vi "main(Test DQMH modules).vi"() -> ()   [LabVIEW 2018, in "Application.lvlib"] (continued)
        n1221 = Build Array("Test DRV 31", "Test DRV 32", "Test DRV 33", "Test DRV 34", "Test DRV 35", "Test DRV 36", "MEAS.requestAC") -> (w2868:string[])
        n1222 = Reverse 1D Array(array=w2868) -> (reversed array=w2869:string[])
        n1223 = for {
          tunnel: w2869 -> [w2903] mode=indexing
          tunnel: [w2902] -> w2860 mode=indexing
          shift-right: [w2901] -> w2862
          shift-left: w2863 -> [w2904]
          tunnel: w2852 -> [w2900]
          n1224 = call "App enquece.vi"("Priority Enquece"=TRUE, "error in (no error)"=w2900, "command"=w2903, "queue in"=w2904) -> ("error out"=w2902:errorcluster, "Queue out"=w2901:refnum<queue>)  [unwired: 6 in]
        }
        n1225 = Initialize Array(TRUE, 6 ("dimension size")) -> (w2880:bool[])
        n1226 = Merge Errors(w2860) -> (w2859:errorcluster)
        n1227 = To Variant(anything=T5."mux10_1_channel6" ("mux10_1(x6)_encode")) -> (Variant=w2889:variant)
        n1228 = To Variant(anything=T6."demux1_10_channel6" ("demux1_10(x6)_encode")) -> (Variant=w2885:variant)
        n1229 = To Variant(anything=w2880) -> (Variant=w2879:variant)
        n1230 = Bundle By Name(cluster=w2877, "command"="MEAS.mux10-1", "command data"=w2889) -> (w2884:T11)
        n1231 = Bundle By Name(cluster=w2877, "command"="MEAS.demux1-10", "command data"=w2885) -> (w2883:T11)
        n1232 = Bundle By Name(cluster=w2877, "command"="MEAS.eMIC", "command data"=w2879) -> (w2878:T11)
        n1233 = Build Array(w2884, w2883, w2878) -> (w2858:T11[])
        n1234 = Reverse 1D Array(array=w2858) -> (reversed array=w2857:T11[])
        n1235 = for {
          tunnel: w2857 -> [w2915] mode=indexing
          tunnel: [w2912] -> w2870 mode=indexing
          tunnel: w2859 -> [w2911]
          tunnel: w2862 -> [w2916]
          n1236 = Unbundle By Name(w2915) -> ("command"=w2914:string, "command data"=w2913:variant)
          n1237 = call "App enquece.vi"("Priority Enquece"=TRUE, "error in (no error)"=w2911, "command data"=w2913, "command"=w2914, "queue in"=w2916) -> ("error out"=w2912:errorcluster)  [unwired: 5 in, 1 out]
        }
        n1238 = Merge Errors(w2873, w2870) -> (w2874:errorcluster)
      }
      frame "Test Channel 7" {
        w2947 = 7  # DUT channel (1-11)
        w2948 = T11 {"command"="", "command data"=variant} ("element")
        n1239 = disable-structure shown="LOGGING==TRUE" {
          disable-tunnel: w2942 -> [w2977 _]
          frame condition #0 (active) {
            n1240 = Empty String/Path?(string/path=w2977) -> (empty?=w2980:bool)
            n1241 = Select(t="Quece timeout", s=w2980, f=w2977) -> (s? t:f=w2976:string)
            n1242 = call "string log (SubVI).vi"("Enum"=enum16{"Init", "Log", "Read"}."Log", "state Name"=w2976) -> ()  [unwired: 8 in, 2 out]
          }
          frame condition #1 {
          }
        }
        n1243 = Build Array("Apps.UI Update", "MEAS.AllRelaysOFF2", "Apps.WaitForEvent") -> (w2926:string[])
        n1244 = for {
          tunnel: [w2967] -> w2933 mode=indexing
          shift-right: [w2968] -> w2934
          shift-left: w2929 -> [w2966]
          tunnel: w2926 -> [w2965] mode=indexing
          n1245 = call "App enquece.vi"("Priority Enquece"=TRUE, "command"=w2965, "queue in"=w2966) -> ("error out"=w2967:errorcluster, "Queue out"=w2968:refnum<queue>)  [unwired: 7 in]
        }
        n1246 = Merge Errors(w2933) -> (w2925:errorcluster)
        n1247 = Build Array("Test DRV 37", "Test DRV 38", "Test DRV 39", "Test DRV 40", "Test DRV 41", "Test DRV 42", "MEAS.requestAC") -> (w2939:string[])
        n1248 = Reverse 1D Array(array=w2939) -> (reversed array=w2940:string[])
        n1249 = for {
          tunnel: w2940 -> [w2974] mode=indexing
          tunnel: [w2973] -> w2932 mode=indexing
          shift-right: [w2972] -> w2924
          shift-left: w2934 -> [w2975]
          tunnel: w2925 -> [w2971]
          n1250 = call "App enquece.vi"("Priority Enquece"=TRUE, "error in (no error)"=w2971, "command"=w2974, "queue in"=w2975) -> ("error out"=w2973:errorcluster, "Queue out"=w2972:refnum<queue>)  [unwired: 6 in]
        }
        n1251 = Merge Errors(w2932) -> (w2931:errorcluster)
        n1252 = Initialize Array(TRUE, 6 ("dimension size")) -> (w2951:bool[])
        n1253 = To Variant(anything=w2951) -> (Variant=w2950:variant)
        n1254 = To Variant(anything=T5."mux10_1_channel7" ("mux10_1(x6)_encode")) -> (Variant=w2960:variant)
        n1255 = To Variant(anything=T6."demux1_10_channel7" ("demux1_10(x6)_encode")) -> (Variant=w2956:variant)
        n1256 = Bundle By Name(cluster=w2948, "command"="MEAS.mux10-1", "command data"=w2960) -> (w2955:T11)
        n1257 = Bundle By Name(cluster=w2948, "command"="MEAS.demux1-10", "command data"=w2956) -> (w2954:T11)
        n1258 = Bundle By Name(cluster=w2948, "command"="MEAS.eMIC", "command data"=w2950) -> (w2949:T11)
        n1259 = Build Array(w2955, w2954, w2949) -> (w2930:T11[])
        n1260 = Reverse 1D Array(array=w2930) -> (reversed array=w2923:T11[])
        n1261 = for {
          tunnel: w2923 -> [w2987] mode=indexing
          tunnel: [w2984] -> w2941 mode=indexing
          tunnel: w2931 -> [w2983]
          tunnel: w2924 -> [w2981]
          n1262 = Unbundle By Name(w2987) -> ("command"=w2986:string, "command data"=w2985:variant)
          n1263 = call "App enquece.vi"("Priority Enquece"=TRUE, "error in (no error)"=w2983, "command data"=w2985, "command"=w2986, "queue in"=w2981) -> ("error out"=w2984:errorcluster)  [unwired: 5 in, 1 out]
        }
        n1264 = Merge Errors(w2944, w2941) -> (w2945:errorcluster)
      }
      frame "Test Channel 8" {
        w3018 = 8  # DUT channel (1-11)
        w3019 = T11 {"command"="", "command data"=variant} ("element")
        n1265 = disable-structure shown="LOGGING==TRUE" {
          disable-tunnel: w3013 -> [w3048 _]
          frame condition #0 (active) {
            n1266 = Empty String/Path?(string/path=w3048) -> (empty?=w3051:bool)
            n1267 = Select(t="Quece timeout", s=w3051, f=w3048) -> (s? t:f=w3047:string)
            n1268 = call "string log (SubVI).vi"("Enum"=enum16{"Init", "Log", "Read"}."Log", "state Name"=w3047) -> ()  [unwired: 8 in, 2 out]
          }
          frame condition #1 {
          }
        }
        n1269 = Build Array("Apps.UI Update", "MEAS.AllRelaysOFF2", "Apps.WaitForEvent") -> (w2997:string[])
        n1270 = for {
          tunnel: [w3038] -> w3005 mode=indexing
          shift-right: [w3039] -> w3007
          shift-left: w3000 -> [w3037]
          tunnel: w2997 -> [w3036] mode=indexing
          n1271 = call "App enquece.vi"("Priority Enquece"=TRUE, "command"=w3036, "queue in"=w3037) -> ("error out"=w3038:errorcluster, "Queue out"=w3039:refnum<queue>)  [unwired: 7 in]
        }
        n1272 = Merge Errors(w3005) -> (w2996:errorcluster)
        n1273 = Build Array("Test DRV 43", "Test DRV 44", "Test DRV 45", "Test DRV 46", "Test DRV 47", "Test DRV 48", "MEAS.requestAC") -> (w3010:string[])
        n1274 = Reverse 1D Array(array=w3010) -> (reversed array=w3011:string[])
        n1275 = for {
          tunnel: w3011 -> [w3045] mode=indexing
          tunnel: [w3044] -> w3004 mode=indexing
          shift-right: [w3043] -> w3006
          shift-left: w3007 -> [w3046]
          tunnel: w2996 -> [w3042]
          n1276 = call "App enquece.vi"("Priority Enquece"=TRUE, "error in (no error)"=w3042, "command"=w3045, "queue in"=w3046) -> ("error out"=w3044:errorcluster, "Queue out"=w3043:refnum<queue>)  [unwired: 6 in]
        }
        n1277 = Initialize Array(TRUE, 6 ("dimension size")) -> (w3022:bool[])
        n1278 = Merge Errors(w3004) -> (w3003:errorcluster)
        n1279 = To Variant(anything=T5."mux10_1_channel8" ("mux10_1(x6)_encode")) -> (Variant=w3031:variant)
        n1280 = To Variant(anything=T6."demux1_10_channel8" ("demux1_10(x6)_encode")) -> (Variant=w3027:variant)
        n1281 = To Variant(anything=w3022) -> (Variant=w3021:variant)
        n1282 = Bundle By Name(cluster=w3019, "command"="MEAS.mux10-1", "command data"=w3031) -> (w3026:T11)
        n1283 = Bundle By Name(cluster=w3019, "command"="MEAS.demux1-10", "command data"=w3027) -> (w3025:T11)
        n1284 = Bundle By Name(cluster=w3019, "command"="MEAS.eMIC", "command data"=w3021) -> (w3020:T11)
        n1285 = Build Array(w3026, w3025, w3020) -> (w3002:T11[])
        n1286 = Reverse 1D Array(array=w3002) -> (reversed array=w3001:T11[])
        n1287 = for {
          tunnel: w3001 -> [w3057] mode=indexing
          tunnel: [w3054] -> w3012 mode=indexing
          tunnel: w3003 -> [w3053]
          tunnel: w3006 -> [w3058]
          n1288 = Unbundle By Name(w3057) -> ("command"=w3056:string, "command data"=w3055:variant)
          n1289 = call "App enquece.vi"("Priority Enquece"=TRUE, "error in (no error)"=w3053, "command data"=w3055, "command"=w3056, "queue in"=w3058) -> ("error out"=w3054:errorcluster)  [unwired: 5 in, 1 out]
        }
        n1290 = Merge Errors(w3015, w3012) -> (w3016:errorcluster)
      }
      frame "Test Channel 9" {
        w3090 = 9  # DUT channel (1-10)
        w3091 = T11 {"command"="", "command data"=variant} ("element")
        n1291 = disable-structure shown="LOGGING==TRUE" {
          disable-tunnel: w3085 -> [w3119 _]
          frame condition #0 (active) {
            n1292 = Empty String/Path?(string/path=w3119) -> (empty?=w3122:bool)
            n1293 = Select(t="Quece timeout", s=w3122, f=w3119) -> (s? t:f=w3118:string)
            n1294 = call "string log (SubVI).vi"("Enum"=enum16{"Init", "Log", "Read"}."Log", "state Name"=w3118) -> ()  [unwired: 8 in, 2 out]
          }
          frame condition #1 {
          }
        }
        n1295 = Build Array("Apps.UI Update", "MEAS.AllRelaysOFF2", "Apps.WaitForEvent") -> (w3067:string[])
        n1296 = for {
          tunnel: [w3109] -> w3076 mode=indexing
          shift-right: [w3110] -> w3078
          shift-left: w3071 -> [w3108]
          tunnel: w3067 -> [w3107] mode=indexing
          n1297 = call "App enquece.vi"("Priority Enquece"=TRUE, "command"=w3107, "queue in"=w3108) -> ("error out"=w3109:errorcluster, "Queue out"=w3110:refnum<queue>)  [unwired: 7 in]
        }
        n1298 = Merge Errors(w3076) -> (w3066:errorcluster)
        n1299 = Build Array("Test DRV 49", "Test DRV 50", "Test DRV 51", "Test DRV 52", "Test DRV 53", "Test DRV 54", "MEAS.requestAC") -> (w3082:string[])
        n1300 = Reverse 1D Array(array=w3082) -> (reversed array=w3083:string[])
        n1301 = for {
          tunnel: w3083 -> [w3116] mode=indexing
          tunnel: [w3115] -> w3075 mode=indexing
          shift-right: [w3114] -> w3077
          shift-left: w3078 -> [w3117]
          tunnel: w3066 -> [w3113]
          n1302 = call "App enquece.vi"("Priority Enquece"=TRUE, "error in (no error)"=w3113, "command"=w3116, "queue in"=w3117) -> ("error out"=w3115:errorcluster, "Queue out"=w3114:refnum<queue>)  [unwired: 6 in]
        }
        n1303 = Merge Errors(w3075) -> (w3074:errorcluster)
        n1304 = Initialize Array(TRUE, 6 ("dimension size")) -> (w3094:bool[])
        n1305 = To Variant(anything=T5."mux10_1_channel9" ("mux10_1(x6)_encode")) -> (Variant=w3103:variant)
        n1306 = To Variant(anything=T6."demux1_10_channel9" ("demux1_10(x6)_encode")) -> (Variant=w3099:variant)
        n1307 = To Variant(anything=w3094) -> (Variant=w3093:variant)
        n1308 = Bundle By Name(cluster=w3091, "command"="MEAS.mux10-1", "command data"=w3103) -> (w3098:T11)
        n1309 = Bundle By Name(cluster=w3091, "command"="MEAS.demux1-10", "command data"=w3099) -> (w3097:T11)
        n1310 = Bundle By Name(cluster=w3091, "command"="MEAS.eMIC", "command data"=w3093) -> (w3092:T11)
        n1311 = Build Array(w3098, w3097, w3092) -> (w3073:T11[])
        n1312 = Reverse 1D Array(array=w3073) -> (reversed array=w3072:T11[])
        n1313 = for {
          tunnel: w3072 -> [w3128] mode=indexing
          tunnel: [w3125] -> w3084 mode=indexing
          tunnel: w3074 -> [w3124]
          tunnel: w3077 -> [w3129]
          n1314 = Unbundle By Name(w3128) -> ("command"=w3127:string, "command data"=w3126:variant)
          n1315 = call "App enquece.vi"("Priority Enquece"=TRUE, "error in (no error)"=w3124, "command data"=w3126, "command"=w3127, "queue in"=w3129) -> ("error out"=w3125:errorcluster)  [unwired: 5 in, 1 out]
        }
        n1316 = Merge Errors(w3087, w3084) -> (w3088:errorcluster)
      }
      frame "Test Channel 10" {
        w3163 = 10  # DUT channel (1-10)
        w3139 = T11 {"command"="", "command data"=variant} ("element")
        n1317 = disable-structure shown="LOGGING==TRUE" {
          disable-tunnel: w3158 -> [w3190 _]
          frame condition #0 (active) {
            n1318 = Empty String/Path?(string/path=w3190) -> (empty?=w3193:bool)
            n1319 = Select(t="Quece timeout", s=w3193, f=w3190) -> (s? t:f=w3189:string)
            n1320 = call "string log (SubVI).vi"("Enum"=enum16{"Init", "Log", "Read"}."Log", "state Name"=w3189) -> ()  [unwired: 8 in, 2 out]
          }
          frame condition #1 {
          }
        }
        n1321 = Build Array("Apps.UI Update", "MEAS.AllRelaysOFF2", "Apps.WaitForEvent") -> (w3141:string[])
        n1322 = for {
          tunnel: [w3180] -> w3149 mode=indexing
          shift-right: [w3181] -> w3151
          shift-left: w3144 -> [w3179]
          tunnel: w3141 -> [w3178] mode=indexing
          n1323 = call "App enquece.vi"("Priority Enquece"=TRUE, "command"=w3178, "queue in"=w3179) -> ("error out"=w3180:errorcluster, "Queue out"=w3181:refnum<queue>)  [unwired: 7 in]
        }
        n1324 = Merge Errors(w3149) -> (w3140:errorcluster)
        n1325 = Build Array("Test DRV 55", "Test DRV 56", "Test DRV 57", "Test DRV 58", "Test DRV 59", "Test DRV 60", "MEAS.requestAC") -> (w3155:string[])
        n1326 = Reverse 1D Array(array=w3155) -> (reversed array=w3156:string[])
        n1327 = for {
          tunnel: w3156 -> [w3187] mode=indexing
          tunnel: [w3186] -> w3148 mode=indexing
          shift-right: [w3185] -> w3150
          shift-left: w3151 -> [w3188]
          tunnel: w3140 -> [w3184]
          n1328 = call "App enquece.vi"("Priority Enquece"=TRUE, "error in (no error)"=w3184, "command"=w3187, "queue in"=w3188) -> ("error out"=w3186:errorcluster, "Queue out"=w3185:refnum<queue>)  [unwired: 6 in]
        }
        n1329 = Initialize Array(TRUE, 6 ("dimension size")) -> (w3133:bool[])
        n1330 = To Variant(anything=w3133) -> (Variant=w3165:variant)
        n1331 = To Variant(anything=T5."mux10_1_channel10" ("mux10_1(x6)_encode")) -> (Variant=w3173:variant)
        n1332 = To Variant(anything=T6."demux1_10_channel10" ("demux1_10(x6)_encode")) -> (Variant=w3169:variant)
        n1333 = Bundle By Name(cluster=w3139, "command"="MEAS.mux10-1", "command data"=w3173) -> (w3168:T11)
        n1334 = Bundle By Name(cluster=w3139, "command"="MEAS.demux1-10", "command data"=w3169) -> (w3167:T11)
        n1335 = Bundle By Name(cluster=w3139, "command"="MEAS.eMIC", "command data"=w3165) -> (w3164:T11)
        n1336 = Merge Errors(w3148) -> (w3147:errorcluster)
        n1337 = Build Array(w3168, w3167, w3164) -> (w3146:T11[])
        n1338 = Reverse 1D Array(array=w3146) -> (reversed array=w3145:T11[])
        n1339 = for {
          tunnel: w3145 -> [w3199] mode=indexing
          tunnel: [w3196] -> w3157 mode=indexing
          tunnel: w3147 -> [w3195]
          tunnel: w3150 -> [w3200]
          n1340 = Unbundle By Name(w3199) -> ("command"=w3198:string, "command data"=w3197:variant)
          n1341 = call "App enquece.vi"("Priority Enquece"=TRUE, "error in (no error)"=w3195, "command data"=w3197, "command"=w3198, "queue in"=w3200) -> ("error out"=w3196:errorcluster)  [unwired: 5 in, 1 out]
        }
        n1342 = Merge Errors(w3160, w3157) -> (w3161:errorcluster)
      }
      frame "Test Channel 10A" {
        w3211 = T11 {"command"="", "command data"=variant} ("element")
        w3239 = 10  # DUT channel (1-10)
        w3219 = T11 {"command"="", "command data"=variant} ("element")
        n1343 = disable-structure shown="LOGGING==TRUE" {
          disable-tunnel: w3234 -> [w3268 _]
          frame condition #0 (active) {
            n1344 = Empty String/Path?(string/path=w3268) -> (empty?=w3271:bool)
            n1345 = Select(t="Quece timeout", s=w3271, f=w3268) -> (s? t:f=w3267:string)
            n1346 = call "string log (SubVI).vi"("Enum"=enum16{"Init", "Log", "Read"}."Log", "state Name"=w3267) -> ()  [unwired: 8 in, 2 out]
          }
          frame condition #1 {
          }
        }
        n1347 = Bundle By Name(cluster=w3211, "command"="Apps.UI Update", "command data"="A") -> (w3210:T11)
        n1348 = Bundle By Name(cluster=w3211, "command"="MEAS.AllRelaysOFF2") -> (w3209:T11)
        n1349 = Bundle By Name(cluster=w3211, "command"="Apps.WaitForEvent") -> (w3208:T11)
        n1350 = Build Array(w3210, w3209, w3208) -> (w3221:T11[])
        n1351 = for {
          tunnel: [w3258] -> w3228 mode=indexing
          shift-right: [w3259] -> w3230
          shift-left: w3223 -> [w3257]
          tunnel: w3221 -> [w3256] mode=indexing
          n1352 = Unbundle By Name(w3256) -> ("command"=w3255:string, "command data"=w3254:variant)
          n1353 = call "App enquece.vi"("Priority Enquece"=TRUE, "command data"=w3254, "command"=w3255, "queue in"=w3257) -> ("error out"=w3258:errorcluster, "Queue out"=w3259:refnum<queue>)  [unwired: 6 in]
        }
        n1354 = Merge Errors(w3228) -> (w3220:errorcluster)
        n1355 = Build Array("Test DRV 55", "WaitFor", "MEAS.requestAC") -> (w3231:string[])
        n1356 = Reverse 1D Array(array=w3231) -> (reversed array=w3232:string[])
        n1357 = for {
          tunnel: w3232 -> [w3265] mode=indexing
          tunnel: [w3264] -> w3227 mode=indexing
          shift-right: [w3263] -> w3229
          shift-left: w3230 -> [w3266]
          tunnel: w3220 -> [w3262]
          n1358 = call "App enquece.vi"("Priority Enquece"=TRUE, "error in (no error)"=w3262, "command"=w3265, "queue in"=w3266) -> ("error out"=w3264:errorcluster, "Queue out"=w3263:refnum<queue>)  [unwired: 6 in]
        }
        n1359 = Initialize Array(FALSE ("element"), 6 ("dimension size")) -> (w3205:bool[])
        n1360 = Initialize Array(TRUE, 1 ("dimension size")) -> (w3204:bool[])
        n1361 = Replace Array Subset(array=w3205, new element=w3204) -> (w3203:bool[])  [unwired: 1 in]
        n1362 = To Variant(anything=T5."mux10_1_channel10" ("mux10_1(x6)_encode")) -> (Variant=w3249:variant)
        n1363 = To Variant(anything=T6."demux1_10_channel10" ("demux1_10(x6)_encode")) -> (Variant=w3245:variant)
        n1364 = To Variant(anything=w3203) -> (Variant=w3241:variant)
        n1365 = Merge Errors(w3227) -> (w3226:errorcluster)
        n1366 = Bundle By Name(cluster=w3219, "command"="MEAS.mux10-1", "command data"=w3249) -> (w3244:T11)
        n1367 = Bundle By Name(cluster=w3219, "command"="MEAS.demux1-10", "command data"=w3245) -> (w3243:T11)
        n1368 = Bundle By Name(cluster=w3219, "command"="MEAS.eMIC", "command data"=w3241) -> (w3240:T11)
        n1369 = Build Array(w3244, w3243, w3240) -> (w3225:T11[])
        n1370 = Reverse 1D Array(array=w3225) -> (reversed array=w3224:T11[])
        n1371 = for {
          tunnel: w3224 -> [w3277] mode=indexing
          tunnel: [w3274] -> w3233 mode=indexing
          tunnel: w3226 -> [w3273]
          tunnel: w3229 -> [w3278]
          n1372 = Unbundle By Name(w3277) -> ("command"=w3276:string, "command data"=w3275:variant)
          n1373 = call "App enquece.vi"("Priority Enquece"=TRUE, "error in (no error)"=w3273, "command data"=w3275, "command"=w3276, "queue in"=w3278) -> ("error out"=w3274:errorcluster)  [unwired: 5 in, 1 out]
        }
        n1374 = Merge Errors(w3236, w3233) -> (w3237:errorcluster)
      }
      frame "Test Channel 10B" {
        w3289 = T11 {"command"="", "command data"=variant} ("element")
        w3318 = 10  # DUT channel (1-10)
        w3297 = T11 {"command"="", "command data"=variant} ("element")
        n1375 = disable-structure shown="LOGGING==TRUE" {
          disable-tunnel: w3313 -> [w3347 _]
          frame condition #0 (active) {
            n1376 = Empty String/Path?(string/path=w3347) -> (empty?=w3350:bool)
            n1377 = Select(t="Quece timeout", s=w3350, f=w3347) -> (s? t:f=w3346:string)
            n1378 = call "string log (SubVI).vi"("Enum"=enum16{"Init", "Log", "Read"}."Log", "state Name"=w3346) -> ()  [unwired: 8 in, 2 out]
          }
          frame condition #1 {
          }
        }
        n1379 = Bundle By Name(cluster=w3289, "command"="Apps.UI Update", "command data"="B") -> (w3288:T11)
        n1380 = Bundle By Name(cluster=w3289, "command"="MEAS.AllRelaysOFF2") -> (w3287:T11)
        n1381 = Bundle By Name(cluster=w3289, "command"="Apps.WaitForEvent") -> (w3286:T11)
        n1382 = Build Array(w3288, w3287, w3286) -> (w3299:T11[])
        n1383 = for {
          tunnel: [w3337] -> w3306 mode=indexing
          shift-right: [w3338] -> w3308
          shift-left: w3301 -> [w3336]
          tunnel: w3299 -> [w3335] mode=indexing
          n1384 = Unbundle By Name(w3335) -> ("command"=w3334:string, "command data"=w3333:variant)
          n1385 = call "App enquece.vi"("Priority Enquece"=TRUE, "command data"=w3333, "command"=w3334, "queue in"=w3336) -> ("error out"=w3337:errorcluster, "Queue out"=w3338:refnum<queue>)  [unwired: 6 in]
        }
        n1386 = Merge Errors(w3306) -> (w3298:errorcluster)
        n1387 = Build Array("Test DRV 55", "Test DRV 56", "WaitFor", "MEAS.requestAC") -> (w3310:string[])
        n1388 = Reverse 1D Array(array=w3310) -> (reversed array=w3311:string[])
        n1389 = for {
          tunnel: w3311 -> [w3344] mode=indexing
          tunnel: [w3343] -> w3305 mode=indexing
          shift-right: [w3342] -> w3307
          shift-left: w3308 -> [w3345]
          tunnel: w3298 -> [w3341]
          n1390 = call "App enquece.vi"("Priority Enquece"=TRUE, "error in (no error)"=w3341, "command"=w3344, "queue in"=w3345) -> ("error out"=w3343:errorcluster, "Queue out"=w3342:refnum<queue>)  [unwired: 6 in]
        }
        n1391 = Initialize Array(FALSE ("element"), 6 ("dimension size")) -> (w3281:bool[])
        n1392 = Initialize Array(TRUE, 2 ("dimension size")) -> (w3280:bool[])
        n1393 = Replace Array Subset(array=w3281, new element=w3280) -> (w3279:bool[])  [unwired: 1 in]
        n1394 = To Variant(anything=T5."mux10_1_channel10" ("mux10_1(x6)_encode")) -> (Variant=w3328:variant)
        n1395 = To Variant(anything=T6."demux1_10_channel10" ("demux1_10(x6)_encode")) -> (Variant=w3324:variant)
        n1396 = To Variant(anything=w3279) -> (Variant=w3320:variant)
        n1397 = Merge Errors(w3305) -> (w3304:errorcluster)
        n1398 = Bundle By Name(cluster=w3297, "command"="MEAS.mux10-1", "command data"=w3328) -> (w3323:T11)
        n1399 = Bundle By Name(cluster=w3297, "command"="MEAS.demux1-10", "command data"=w3324) -> (w3322:T11)
        n1400 = Bundle By Name(cluster=w3297, "command"="MEAS.eMIC", "command data"=w3320) -> (w3319:T11)
        n1401 = Build Array(w3323, w3322, w3319) -> (w3303:T11[])
        n1402 = Reverse 1D Array(array=w3303) -> (reversed array=w3302:T11[])
        n1403 = for {
          tunnel: w3302 -> [w3356] mode=indexing
          tunnel: [w3353] -> w3312 mode=indexing
          tunnel: w3304 -> [w3352]
          tunnel: w3307 -> [w3357]
          n1404 = Unbundle By Name(w3356) -> ("command"=w3355:string, "command data"=w3354:variant)
          n1405 = call "App enquece.vi"("Priority Enquece"=TRUE, "error in (no error)"=w3352, "command data"=w3354, "command"=w3355, "queue in"=w3357) -> ("error out"=w3353:errorcluster)  [unwired: 5 in, 1 out]
        }
        n1406 = Merge Errors(w3315, w3312) -> (w3316:errorcluster)
      }
      frame "Test Channel 10C" {
        w3371 = T11 {"command"="", "command data"=variant} ("element")
        w3398 = 10  # DUT channel (1-10)
        w3378 = T11 {"command"="", "command data"=variant} ("element")
        n1407 = disable-structure shown="LOGGING==TRUE" {
          disable-tunnel: w3393 -> [w3427 _]
          frame condition #0 (active) {
            n1408 = Empty String/Path?(string/path=w3427) -> (empty?=w3430:bool)
            n1409 = Select(t="Quece timeout", s=w3430, f=w3427) -> (s? t:f=w3426:string)
            n1410 = call "string log (SubVI).vi"("Enum"=enum16{"Init", "Log", "Read"}."Log", "state Name"=w3426) -> ()  [unwired: 8 in, 2 out]
          }
          frame condition #1 {
          }
        }
        n1411 = Bundle By Name(cluster=w3371, "command"="Apps.UI Update", "command data"="C") -> (w3370:T11)
        n1412 = Bundle By Name(cluster=w3371, "command"="MEAS.AllRelaysOFF2") -> (w3369:T11)
        n1413 = Bundle By Name(cluster=w3371, "command"="Apps.WaitForEvent") -> (w3368:T11)
        n1414 = Build Array(w3370, w3369, w3368) -> (w3380:T11[])
        n1415 = for {
          tunnel: [w3417] -> w3387 mode=indexing
          shift-right: [w3418] -> w3389
          shift-left: w3382 -> [w3416]
          tunnel: w3380 -> [w3415] mode=indexing
          n1416 = Unbundle By Name(w3415) -> ("command"=w3414:string, "command data"=w3413:variant)
          n1417 = call "App enquece.vi"("Priority Enquece"=TRUE, "command data"=w3413, "command"=w3414, "queue in"=w3416) -> ("error out"=w3417:errorcluster, "Queue out"=w3418:refnum<queue>)  [unwired: 6 in]
        }
        n1418 = Merge Errors(w3387) -> (w3379:errorcluster)
        n1419 = Build Array("Test DRV 55", "Test DRV 56", "Test DRV 57", "WaitFor", "MEAS.requestAC") -> (w3390:string[])
        n1420 = Reverse 1D Array(array=w3390) -> (reversed array=w3391:string[])
        n1421 = for {
          tunnel: w3391 -> [w3424] mode=indexing
          tunnel: [w3423] -> w3386 mode=indexing
          shift-right: [w3422] -> w3388
          shift-left: w3389 -> [w3425]
          tunnel: w3379 -> [w3421]
          n1422 = call "App enquece.vi"("Priority Enquece"=TRUE, "error in (no error)"=w3421, "command"=w3424, "queue in"=w3425) -> ("error out"=w3423:errorcluster, "Queue out"=w3422:refnum<queue>)  [unwired: 6 in]
        }
        n1423 = Initialize Array(FALSE ("element"), 6 ("dimension size")) -> (w3363:bool[])
        n1424 = Initialize Array(TRUE, 3 ("dimension size")) -> (w3362:bool[])
        n1425 = Replace Array Subset(array=w3363, new element=w3362) -> (w3361:bool[])  [unwired: 1 in]
        n1426 = To Variant(anything=T5."mux10_1_channel10" ("mux10_1(x6)_encode")) -> (Variant=w3408:variant)
        n1427 = To Variant(anything=T6."demux1_10_channel10" ("demux1_10(x6)_encode")) -> (Variant=w3404:variant)
        n1428 = To Variant(anything=w3361) -> (Variant=w3400:variant)
        n1429 = Merge Errors(w3386) -> (w3385:errorcluster)
        n1430 = Bundle By Name(cluster=w3378, "command"="MEAS.mux10-1", "command data"=w3408) -> (w3403:T11)
        n1431 = Bundle By Name(cluster=w3378, "command"="MEAS.demux1-10", "command data"=w3404) -> (w3402:T11)
        n1432 = Bundle By Name(cluster=w3378, "command"="MEAS.eMIC", "command data"=w3400) -> (w3399:T11)
        n1433 = Build Array(w3403, w3402, w3399) -> (w3384:T11[])
        n1434 = Reverse 1D Array(array=w3384) -> (reversed array=w3383:T11[])
        n1435 = for {
          tunnel: w3383 -> [w3436] mode=indexing
          tunnel: [w3433] -> w3392 mode=indexing
          tunnel: w3385 -> [w3432]
          tunnel: w3388 -> [w3437]
          n1436 = Unbundle By Name(w3436) -> ("command"=w3435:string, "command data"=w3434:variant)
          n1437 = call "App enquece.vi"("Priority Enquece"=TRUE, "error in (no error)"=w3432, "command data"=w3434, "command"=w3435, "queue in"=w3437) -> ("error out"=w3433:errorcluster)  [unwired: 5 in, 1 out]
        }
        n1438 = Merge Errors(w3395, w3392) -> (w3396:errorcluster)
      }
      frame "Test Channel 10D" {
        w3452 = T11 {"command"="", "command data"=variant} ("element")
        w3479 = 10  # DUT channel (1-10)
        w3459 = T11 {"command"="", "command data"=variant} ("element")
        n1439 = disable-structure shown="LOGGING==TRUE" {
          disable-tunnel: w3474 -> [w3508 _]
          frame condition #0 (active) {
            n1440 = Empty String/Path?(string/path=w3508) -> (empty?=w3511:bool)
            n1441 = Select(t="Quece timeout", s=w3511, f=w3508) -> (s? t:f=w3507:string)
            n1442 = call "string log (SubVI).vi"("Enum"=enum16{"Init", "Log", "Read"}."Log", "state Name"=w3507) -> ()  [unwired: 8 in, 2 out]
          }
          frame condition #1 {
          }
        }
        n1443 = Bundle By Name(cluster=w3452, "command"="Apps.UI Update", "command data"="D") -> (w3451:T11)
        n1444 = Bundle By Name(cluster=w3452, "command"="MEAS.AllRelaysOFF2") -> (w3450:T11)
        n1445 = Bundle By Name(cluster=w3452, "command"="Apps.WaitForEvent") -> (w3449:T11)
        n1446 = Build Array(w3451, w3450, w3449) -> (w3461:T11[])
        n1447 = for {
          tunnel: [w3498] -> w3468 mode=indexing
          shift-right: [w3499] -> w3470
          shift-left: w3463 -> [w3497]
          tunnel: w3461 -> [w3496] mode=indexing
          n1448 = Unbundle By Name(w3496) -> ("command"=w3495:string, "command data"=w3494:variant)
          n1449 = call "App enquece.vi"("Priority Enquece"=TRUE, "command data"=w3494, "command"=w3495, "queue in"=w3497) -> ("error out"=w3498:errorcluster, "Queue out"=w3499:refnum<queue>)  [unwired: 6 in]
        }
        n1450 = Merge Errors(w3468) -> (w3460:errorcluster)
        n1451 = Build Array("Test DRV 55", "Test DRV 56", "Test DRV 57", "Test DRV 58", "WaitFor", "MEAS.requestAC") -> (w3471:string[])
        n1452 = Reverse 1D Array(array=w3471) -> (reversed array=w3472:string[])
        n1453 = for {
          tunnel: w3472 -> [w3505] mode=indexing
          tunnel: [w3504] -> w3467 mode=indexing
          shift-right: [w3503] -> w3469
          shift-left: w3470 -> [w3506]
          tunnel: w3460 -> [w3502]
          n1454 = call "App enquece.vi"("Priority Enquece"=TRUE, "error in (no error)"=w3502, "command"=w3505, "queue in"=w3506) -> ("error out"=w3504:errorcluster, "Queue out"=w3503:refnum<queue>)  [unwired: 6 in]
        }
        n1455 = Initialize Array(FALSE ("element"), 6 ("dimension size")) -> (w3444:bool[])
        n1456 = Initialize Array(TRUE, 4 ("dimension size")) -> (w3443:bool[])
        n1457 = Replace Array Subset(array=w3444, new element=w3443) -> (w3442:bool[])  [unwired: 1 in]
        n1458 = To Variant(anything=T5."mux10_1_channel10" ("mux10_1(x6)_encode")) -> (Variant=w3489:variant)
        n1459 = To Variant(anything=T6."demux1_10_channel10" ("demux1_10(x6)_encode")) -> (Variant=w3485:variant)
        n1460 = To Variant(anything=w3442) -> (Variant=w3481:variant)
        n1461 = Merge Errors(w3467) -> (w3466:errorcluster)
        n1462 = Bundle By Name(cluster=w3459, "command"="MEAS.mux10-1", "command data"=w3489) -> (w3484:T11)
        n1463 = Bundle By Name(cluster=w3459, "command"="MEAS.demux1-10", "command data"=w3485) -> (w3483:T11)
        n1464 = Bundle By Name(cluster=w3459, "command"="MEAS.eMIC", "command data"=w3481) -> (w3480:T11)
        n1465 = Build Array(w3484, w3483, w3480) -> (w3465:T11[])
        n1466 = Reverse 1D Array(array=w3465) -> (reversed array=w3464:T11[])
        n1467 = for {
          tunnel: w3464 -> [w3517] mode=indexing
          tunnel: [w3514] -> w3473 mode=indexing
          tunnel: w3466 -> [w3513]
          tunnel: w3469 -> [w3518]
          n1468 = Unbundle By Name(w3517) -> ("command"=w3516:string, "command data"=w3515:variant)
          n1469 = call "App enquece.vi"("Priority Enquece"=TRUE, "error in (no error)"=w3513, "command data"=w3515, "command"=w3516, "queue in"=w3518) -> ("error out"=w3514:errorcluster)  [unwired: 5 in, 1 out]
        }
        n1470 = Merge Errors(w3476, w3473) -> (w3477:errorcluster)
      }
      frame "Test Channel 10E" {
        w3535 = T11 {"command"="", "command data"=variant} ("element")
        w3561 = 10  # DUT channel (1-10)
        w3542 = T11 {"command"="", "command data"=variant} ("element")
        n1471 = disable-structure shown="LOGGING==TRUE" {
          disable-tunnel: w3556 -> [w3590 _]
          frame condition #0 (active) {
            n1472 = Empty String/Path?(string/path=w3590) -> (empty?=w3593:bool)
            n1473 = Select(t="Quece timeout", s=w3593, f=w3590) -> (s? t:f=w3589:string)
            n1474 = call "string log (SubVI).vi"("Enum"=enum16{"Init", "Log", "Read"}."Log", "state Name"=w3589) -> ()  [unwired: 8 in, 2 out]
          }
          frame condition #1 {
          }
        }
        n1475 = Bundle By Name(cluster=w3535, "command"="Apps.UI Update", "command data"="E") -> (w3534:T11)
        n1476 = Bundle By Name(cluster=w3535, "command"="MEAS.AllRelaysOFF2") -> (w3533:T11)
        n1477 = Bundle By Name(cluster=w3535, "command"="Apps.WaitForEvent") -> (w3532:T11)
        n1478 = Build Array(w3534, w3533, w3532) -> (w3544:T11[])
        n1479 = for {
          tunnel: [w3580] -> w3551 mode=indexing
          shift-right: [w3581] -> w3553
          shift-left: w3546 -> [w3579]
          tunnel: w3544 -> [w3578] mode=indexing
          n1480 = Unbundle By Name(w3578) -> ("command"=w3577:string, "command data"=w3576:variant)
          n1481 = call "App enquece.vi"("Priority Enquece"=TRUE, "command data"=w3576, "command"=w3577, "queue in"=w3579) -> ("error out"=w3580:errorcluster, "Queue out"=w3581:refnum<queue>)  [unwired: 6 in]
        }
        n1482 = Merge Errors(w3551) -> (w3543:errorcluster)
        n1483 = Build Array("Test DRV 55", "Test DRV 56", "Test DRV 57", "Test DRV 58", "Test DRV 59", "WaitFor", "MEAS.requestAC") -> (w3519:string[])
        n1484 = Reverse 1D Array(array=w3519) -> (reversed array=w3554:string[])
        n1485 = for {
          tunnel: w3554 -> [w3587] mode=indexing
          tunnel: [w3586] -> w3550 mode=indexing
          shift-right: [w3585] -> w3552
          shift-left: w3553 -> [w3588]
          tunnel: w3543 -> [w3584]
          n1486 = call "App enquece.vi"("Priority Enquece"=TRUE, "error in (no error)"=w3584, "command"=w3587, "queue in"=w3588) -> ("error out"=w3586:errorcluster, "Queue out"=w3585:refnum<queue>)  [unwired: 6 in]
        }
        n1487 = Initialize Array(FALSE ("element"), 6 ("dimension size")) -> (w3529:bool[])
        n1488 = Initialize Array(TRUE, 5 ("dimension size")) -> (w3528:bool[])
        n1489 = Replace Array Subset(array=w3529, new element=w3528) -> (w3527:bool[])  [unwired: 1 in]
        n1490 = To Variant(anything=T5."mux10_1_channel10" ("mux10_1(x6)_encode")) -> (Variant=w3571:variant)
        n1491 = To Variant(anything=T6."demux1_10_channel10" ("demux1_10(x6)_encode")) -> (Variant=w3567:variant)
        n1492 = To Variant(anything=w3527) -> (Variant=w3563:variant)
        n1493 = Merge Errors(w3550) -> (w3549:errorcluster)
        n1494 = Bundle By Name(cluster=w3542, "command"="MEAS.mux10-1", "command data"=w3571) -> (w3566:T11)
        n1495 = Bundle By Name(cluster=w3542, "command"="MEAS.demux1-10", "command data"=w3567) -> (w3565:T11)
        n1496 = Bundle By Name(cluster=w3542, "command"="MEAS.eMIC", "command data"=w3563) -> (w3562:T11)
        n1497 = Build Array(w3566, w3565, w3562) -> (w3548:T11[])
        n1498 = Reverse 1D Array(array=w3548) -> (reversed array=w3547:T11[])
        n1499 = for {
          tunnel: w3547 -> [w3599] mode=indexing
          tunnel: [w3596] -> w3555 mode=indexing
          tunnel: w3549 -> [w3595]
          tunnel: w3552 -> [w3600]
          n1500 = Unbundle By Name(w3599) -> ("command"=w3598:string, "command data"=w3597:variant)
          n1501 = call "App enquece.vi"("Priority Enquece"=TRUE, "error in (no error)"=w3595, "command data"=w3597, "command"=w3598, "queue in"=w3600) -> ("error out"=w3596:errorcluster)  [unwired: 5 in, 1 out]
        }
        n1502 = Merge Errors(w3558, w3555) -> (w3559:errorcluster)
      }
      frame "Test DRV 1" {
        w3602 = 1  # DUT index(1-60)
        n1503 = disable-structure shown="LOGGING==TRUE" {
          disable-tunnel: w3606 -> [w3639 _]
          frame condition #0 (active) {
            n1504 = Empty String/Path?(string/path=w3639) -> (empty?=w3642:bool)
            n1505 = Select(t="Quece timeout", s=w3642, f=w3639) -> (s? t:f=w3638:string)
            n1506 = call "string log (SubVI).vi"("Enum"=enum16{"Init", "Log", "Read"}."Log", "state Name"=w3638) -> ()  [unwired: 8 in, 2 out]
          }
          frame condition #1 {
          }
        }
        n1507 = call "progress string(SubVI).vi"("String 3"=w3606, "String in"=w3604) -> ("String out"=w3605:string)  [unwired: 9 in]
        n1508 = call "FGV Driver Data.vi"("DUT index(1-60)"=w3602, "FGV enum(Read)"=FGV_DRV_data."Read" ("FGV enum")) -> ("DUT SC"=w3603:bool)  [unwired: 6 in, 3 out]
        n1509 = case shown="False" w3603 {
          tunnel: [w3631 _] -> w3611
          tunnel: w3608 -> [w3630 _]
          frame False {
            w3618 = T11 {"command"="", "command data"=variant} ("element")
            w3617 = "MEAS.mux6_1"
            n1510 = To Variant(anything=T4."mux6_1_channel1_3" ("mux6_1(3wires)_encode")) -> (Variant=w3628:variant)
            n1511 = To Variant(anything=T4."mux6-1_channel0" ("mux6_1(3wires)_encode")) -> (Variant=w3616:variant)
            n1512 = To Variant(anything=T4."mux6-1_channel1_2" ("mux6_1(3wires)_encode")) -> (Variant=w3626:variant)
            n1513 = Bundle By Name(cluster=w3618, "command"=w3617, "command data"=w3626) -> (w3625:T11)
            n1514 = Bundle By Name(cluster=w3618, "command"=w3617, "command data"=w3628) -> (w3624:T11)
            n1515 = Bundle By Name(cluster=w3618, "command"=w3617, "command data"=w3616) -> ()  [unwired: 1 out]
            n1516 = Bundle By Name(cluster=w3618, "command"="MEAS.DMM dual read") -> (w3622:T11)
            n1517 = Build Array(w3625, w3624, w3622) -> (w3620:T11[])
            n1518 = Reverse 1D Array(array=w3620) -> (reversed array=w3621:T11[])
            n1519 = for {
              tunnel: [w3637] -> w3631 mode=indexing
              tunnel: w3630 -> [w3636]
              tunnel: w3621 -> [w3635] mode=indexing
              n1520 = Unbundle By Name(w3635) -> ("command"=w3634:string, "command data"=w3633:variant)
              n1521 = call "App enquece.vi"("Priority Enquece"=TRUE, "command data"=w3633, "command"=w3634, "queue in"=w3636) -> ("error out"=w3637:errorcluster)  [unwired: 6 in, 1 out]
            }
          }
          frame True {
          }
        }
        n1522 = Merge Errors(w3609, w3611) -> (w3610:errorcluster)
      }
      frame "Test DRV 2" {
        w3644 = 2  # DUT index(1-60)
        n1523 = disable-structure shown="LOGGING==TRUE" {
          disable-tunnel: w3645 -> [w3680 _]
          frame condition #0 (active) {
            n1524 = Empty String/Path?(string/path=w3680) -> (empty?=w3683:bool)
            n1525 = Select(t="Quece timeout", s=w3683, f=w3680) -> (s? t:f=w3679:string)
            n1526 = call "string log (SubVI).vi"("Enum"=enum16{"Init", "Log", "Read"}."Log", "state Name"=w3679) -> ()  [unwired: 8 in, 2 out]
          }
          frame condition #1 {
          }
        }
        n1527 = call "progress string(SubVI).vi"("String 3"=w3645, "String in"=w3646) -> ("String out"=w3647:string)  [unwired: 9 in]
        n1528 = call "FGV Driver Data.vi"("DUT index(1-60)"=w3644) -> ("DUT SC"=w3643:bool)  [unwired: 7 in, 3 out]
        n1529 = case shown="False" w3643 {
          tunnel: [w3672 _] -> w3652
          tunnel: w3649 -> [w3671 _]
          frame False {
            w3657 = T11 {"command"="", "command data"=variant} ("element")
            w3659 = "MEAS.mux6_1"
            n1530 = To Variant(anything=T4."mux6-1_channel0" ("mux6_1(3wires)_encode")) -> (Variant=w3658:variant)
            n1531 = To Variant(anything=T4."mux6_1_channel2_3" ("mux6_1(3wires)_encode")) -> (Variant=w3669:variant)
            n1532 = To Variant(anything=T4."mux6_1_channel2_2" ("mux6_1(3wires)_encode")) -> (Variant=w3667:variant)
            n1533 = Bundle By Name(cluster=w3657, "command"=w3659, "command data"=w3667) -> (w3666:T11)
            n1534 = Bundle By Name(cluster=w3657, "command"=w3659, "command data"=w3669) -> (w3665:T11)
            n1535 = Bundle By Name(cluster=w3657, "command"=w3659, "command data"=w3658) -> ()  [unwired: 1 out]
            n1536 = Bundle By Name(cluster=w3657, "command"="MEAS.DMM dual read") -> (w3663:T11)
            n1537 = Build Array(w3666, w3665, w3663) -> (w3661:T11[])
            n1538 = Reverse 1D Array(array=w3661) -> (reversed array=w3662:T11[])
            n1539 = for {
              tunnel: [w3678] -> w3672 mode=indexing
              tunnel: w3671 -> [w3677]
              tunnel: w3662 -> [w3676] mode=indexing
              n1540 = Unbundle By Name(w3676) -> ("command"=w3675:string, "command data"=w3674:variant)
              n1541 = call "App enquece.vi"("Priority Enquece"=TRUE, "command data"=w3674, "command"=w3675, "queue in"=w3677) -> ("error out"=w3678:errorcluster)  [unwired: 6 in, 1 out]
            }
          }
          frame True {
          }
        }
        n1542 = Merge Errors(w3650, w3652) -> (w3651:errorcluster)
      }
      frame "Test DRV 3" {
        w3685 = 3  # DUT index(1-60)
        n1543 = disable-structure shown="LOGGING==TRUE" {
          disable-tunnel: w3686 -> [w3721 _]
          frame condition #0 (active) {
            n1544 = Empty String/Path?(string/path=w3721) -> (empty?=w3724:bool)
            n1545 = Select(t="Quece timeout", s=w3724, f=w3721) -> (s? t:f=w3720:string)
            n1546 = call "string log (SubVI).vi"("Enum"=enum16{"Init", "Log", "Read"}."Log", "state Name"=w3720) -> ()  [unwired: 8 in, 2 out]
          }
          frame condition #1 {
          }
        }
        n1547 = call "progress string(SubVI).vi"("String 3"=w3686, "String in"=w3687) -> ("String out"=w3688:string)  [unwired: 9 in]
        n1548 = call "FGV Driver Data.vi"("DUT index(1-60)"=w3685) -> ("DUT SC"=w3684:bool)  [unwired: 7 in, 3 out]
        n1549 = case shown="False" w3684 {
          tunnel: [w3713 _] -> w3693
          tunnel: w3690 -> [w3712 _]
          frame False {
            w3700 = T11 {"command"="", "command data"=variant} ("element")
            w3699 = "MEAS.mux6_1"
            n1550 = To Variant(anything=T4."mux6-1_channel0" ("mux6_1(3wires)_encode")) -> (Variant=w3698:variant)
            n1551 = To Variant(anything=T4."mux6_1_channel3_3" ("mux6_1(3wires)_encode")) -> (Variant=w3710:variant)
            n1552 = To Variant(anything=T4."mux6_1_channel3_2" ("mux6_1(3wires)_encode")) -> (Variant=w3708:variant)
            n1553 = Bundle By Name(cluster=w3700, "command"=w3699, "command data"=w3708) -> (w3707:T11)
            n1554 = Bundle By Name(cluster=w3700, "command"=w3699, "command data"=w3710) -> (w3706:T11)
            n1555 = Bundle By Name(cluster=w3700, "command"=w3699, "command data"=w3698) -> ()  [unwired: 1 out]
            n1556 = Bundle By Name(cluster=w3700, "command"="MEAS.DMM dual read") -> (w3704:T11)
            n1557 = Build Array(w3707, w3706, w3704) -> (w3702:T11[])
            n1558 = Reverse 1D Array(array=w3702) -> (reversed array=w3703:T11[])
            n1559 = for {
              tunnel: [w3719] -> w3713 mode=indexing
              tunnel: w3712 -> [w3718]
              tunnel: w3703 -> [w3717] mode=indexing
              n1560 = Unbundle By Name(w3717) -> ("command"=w3716:string, "command data"=w3715:variant)
              n1561 = call "App enquece.vi"("Priority Enquece"=TRUE, "command data"=w3715, "command"=w3716, "queue in"=w3718) -> ("error out"=w3719:errorcluster)  [unwired: 6 in, 1 out]
            }
          }
          frame True {
          }
        }
        n1562 = Merge Errors(w3691, w3693) -> (w3692:errorcluster)
      }
      frame "Test DRV 4" {
        w3726 = 4  # DUT index(0-59)
        n1563 = disable-structure shown="LOGGING==TRUE" {
          disable-tunnel: w3727 -> [w3762 _]
          frame condition #0 (active) {
            n1564 = Empty String/Path?(string/path=w3762) -> (empty?=w3765:bool)
            n1565 = Select(t="Quece timeout", s=w3765, f=w3762) -> (s? t:f=w3761:string)
            n1566 = call "string log (SubVI).vi"("Enum"=enum16{"Init", "Log", "Read"}."Log", "state Name"=w3761) -> ()  [unwired: 8 in, 2 out]
          }
          frame condition #1 {
          }
        }
        n1567 = call "progress string(SubVI).vi"("String 3"=w3727, "String in"=w3728) -> ("String out"=w3729:string)  [unwired: 9 in]
        n1568 = call "FGV Driver Data.vi"("DUT index(1-60)"=w3726) -> ("DUT SC"=w3725:bool)  [unwired: 7 in, 3 out]
        n1569 = case shown="False" w3725 {
          tunnel: [w3754 _] -> w3734
          tunnel: w3731 -> [w3753 _]
          frame False {
            w3741 = T11 {"command"="", "command data"=variant} ("element")
            w3740 = "MEAS.mux6_1"
            n1570 = To Variant(anything=T4."mux6-1_channel0" ("mux6_1(3wires)_encode")) -> (Variant=w3739:variant)
            n1571 = To Variant(anything=T4."mux6_1_channel4_3" ("mux6_1(3wires)_encode")) -> (Variant=w3751:variant)
            n1572 = To Variant(anything=T4."mux6_1_channel4_2" ("mux6_1(3wires)_encode")) -> (Variant=w3749:variant)
            n1573 = Bundle By Name(cluster=w3741, "command"=w3740, "command data"=w3749) -> (w3748:T11)
            n1574 = Bundle By Name(cluster=w3741, "command"=w3740, "command data"=w3751) -> (w3747:T11)
            n1575 = Bundle By Name(cluster=w3741, "command"=w3740, "command data"=w3739) -> ()  [unwired: 1 out]
            n1576 = Bundle By Name(cluster=w3741, "command"="MEAS.DMM dual read") -> (w3745:T11)
            n1577 = Build Array(w3748, w3747, w3745) -> (w3743:T11[])
            n1578 = Reverse 1D Array(array=w3743) -> (reversed array=w3744:T11[])
            n1579 = for {
              tunnel: [w3760] -> w3754 mode=indexing
              tunnel: w3753 -> [w3759]
              tunnel: w3744 -> [w3758] mode=indexing
              n1580 = Unbundle By Name(w3758) -> ("command"=w3757:string, "command data"=w3756:variant)
              n1581 = call "App enquece.vi"("Priority Enquece"=TRUE, "command data"=w3756, "command"=w3757, "queue in"=w3759) -> ("error out"=w3760:errorcluster)  [unwired: 6 in, 1 out]
            }
          }
          frame True {
          }
        }
        n1582 = Merge Errors(w3732, w3734) -> (w3733:errorcluster)
      }
      frame "Test DRV 5" {
        w3767 = 5  # DUT index(0-59)
        n1583 = disable-structure shown="LOGGING==TRUE" {
          disable-tunnel: w3768 -> [w3803 _]
          frame condition #0 (active) {
            n1584 = Empty String/Path?(string/path=w3803) -> (empty?=w3806:bool)
            n1585 = Select(t="Quece timeout", s=w3806, f=w3803) -> (s? t:f=w3802:string)
            n1586 = call "string log (SubVI).vi"("Enum"=enum16{"Init", "Log", "Read"}."Log", "state Name"=w3802) -> ()  [unwired: 8 in, 2 out]
          }
          frame condition #1 {
          }
        }
        n1587 = call "progress string(SubVI).vi"("String 3"=w3768, "String in"=w3769) -> ("String out"=w3770:string)  [unwired: 9 in]
        n1588 = call "FGV Driver Data.vi"("DUT index(1-60)"=w3767) -> ("DUT SC"=w3766:bool)  [unwired: 7 in, 3 out]
        n1589 = case shown="False" w3766 {
          tunnel: [w3795 _] -> w3775
          tunnel: w3772 -> [w3794 _]
          frame False {
            w3782 = T11 {"command"="", "command data"=variant} ("element")
            w3781 = "MEAS.mux6_1"
            n1590 = To Variant(anything=T4."mux6-1_channel0" ("mux6_1(3wires)_encode")) -> (Variant=w3780:variant)
            n1591 = To Variant(anything=T4."mux6_1_channel5_3" ("mux6_1(3wires)_encode")) -> (Variant=w3792:variant)
            n1592 = To Variant(anything=T4."mux6_1_channel5_2" ("mux6_1(3wires)_encode")) -> (Variant=w3790:variant)
            n1593 = Bundle By Name(cluster=w3782, "command"=w3781, "command data"=w3790) -> (w3789:T11)
            n1594 = Bundle By Name(cluster=w3782, "command"=w3781, "command data"=w3792) -> (w3788:T11)
            n1595 = Bundle By Name(cluster=w3782, "command"=w3781, "command data"=w3780) -> ()  [unwired: 1 out]
            n1596 = Bundle By Name(cluster=w3782, "command"="MEAS.DMM dual read") -> (w3786:T11)
            n1597 = Build Array(w3789, w3788, w3786) -> (w3784:T11[])
            n1598 = Reverse 1D Array(array=w3784) -> (reversed array=w3785:T11[])
            n1599 = for {
              tunnel: [w3801] -> w3795 mode=indexing
              tunnel: w3794 -> [w3800]
              tunnel: w3785 -> [w3799] mode=indexing
              n1600 = Unbundle By Name(w3799) -> ("command"=w3798:string, "command data"=w3797:variant)
              n1601 = call "App enquece.vi"("Priority Enquece"=TRUE, "command data"=w3797, "command"=w3798, "queue in"=w3800) -> ("error out"=w3801:errorcluster)  [unwired: 6 in, 1 out]
            }
          }
          frame True {
          }
        }
        n1602 = Merge Errors(w3773, w3775) -> (w3774:errorcluster)
      }
      frame "Test DRV 6" {
        w3811 = 6  # DUT index(0-59)
        n1603 = disable-structure shown="LOGGING==TRUE" {
          disable-tunnel: w3807 -> [w3844 _]
          frame condition #0 (active) {
            n1604 = Empty String/Path?(string/path=w3844) -> (empty?=w3847:bool)
            n1605 = Select(t="Quece timeout", s=w3847, f=w3844) -> (s? t:f=w3843:string)
            n1606 = call "string log (SubVI).vi"("Enum"=enum16{"Init", "Log", "Read"}."Log", "state Name"=w3843) -> ()  [unwired: 8 in, 2 out]
          }
          frame condition #1 {
          }
        }
        n1607 = call "progress string(SubVI).vi"("String 3"=w3807, "String in"=w3808) -> ("String out"=w3809:string)  [unwired: 9 in]
        n1608 = call "FGV Driver Data.vi"("DUT index(1-60)"=w3811) -> ("DUT SC"=w3810:bool)  [unwired: 7 in, 3 out]
        n1609 = case shown="False" w3810 {
          tunnel: [w3836 _] -> w3816
          tunnel: w3813 -> [w3835 _]
          frame False {
            w3823 = T11 {"command"="", "command data"=variant} ("element")
            w3822 = "MEAS.mux6_1"
            n1610 = To Variant(anything=T4."mux6-1_channel0" ("mux6_1(3wires)_encode")) -> (Variant=w3821:variant)
            n1611 = To Variant(anything=T4."mux6_1_channel6_3" ("mux6_1(3wires)_encode")) -> (Variant=w3833:variant)
            n1612 = To Variant(anything=T4."mux6_1_channel6_2" ("mux6_1(3wires)_encode")) -> (Variant=w3831:variant)
            n1613 = Bundle By Name(cluster=w3823, "command"=w3822, "command data"=w3831) -> (w3830:T11)
            n1614 = Bundle By Name(cluster=w3823, "command"=w3822, "command data"=w3833) -> (w3829:T11)
            n1615 = Bundle By Name(cluster=w3823, "command"=w3822, "command data"=w3821) -> ()  [unwired: 1 out]
            n1616 = Bundle By Name(cluster=w3823, "command"="MEAS.DMM dual read") -> (w3827:T11)
            n1617 = Build Array(w3830, w3829, w3827) -> (w3825:T11[])
            n1618 = Reverse 1D Array(array=w3825) -> (reversed array=w3826:T11[])
            n1619 = for {
              tunnel: [w3842] -> w3836 mode=indexing
              tunnel: w3835 -> [w3841]
              tunnel: w3826 -> [w3840] mode=indexing
              n1620 = Unbundle By Name(w3840) -> ("command"=w3839:string, "command data"=w3838:variant)
              n1621 = call "App enquece.vi"("Priority Enquece"=TRUE, "command data"=w3838, "command"=w3839, "queue in"=w3841) -> ("error out"=w3842:errorcluster)  [unwired: 6 in, 1 out]
            }
          }
          frame True {
          }
        }
        n1622 = Merge Errors(w3814, w3816) -> (w3815:errorcluster)
      }
      frame "Test DRV 7" {
        w3849 = 7  # DUT index(0-59)
        n1623 = disable-structure shown="LOGGING==TRUE" {
          disable-tunnel: w3850 -> [w3885 _]
          frame condition #0 (active) {
            n1624 = Empty String/Path?(string/path=w3885) -> (empty?=w3888:bool)
